vi "Constants.vi"() -> ()   [LabVIEW 2015, in "SLSC-12201 DIO Shared.lvlib"]
doc: "Use this Global VI to access the GUIDs assigned to the page resources of the Custom Device."
uses:
  SLSC-12201 DIO Shared.lvlib
panel:
  in  "Tab Control 2":T1(tab)=enum."Properties"
  in  "GUID Line Page":string="661c9457-bca1-4357-942d-be39bffabc16"
  in  "GUID Port Page":string="b5f9d9e4-a9da-4a9f-991b-22d0b235c7c1"
  in  "GUID EnableDisable Page":string="89b0e4bb-853e-450a-b478-3369bedb40c6"
  in  "GUID Command Page":string="5ef2e5ef-6c3e-41ce-8bf3-8b9cdcedadff"
  in  "GUID Status  Page":string="1b9978d0-bb72-4eda-a9bc-ebfaab5f75ec"
  in  "GUID Outgoing Page":string="c55bf871-3108-4625-9a8c-cf5a91b1839b"
  in  "GUID Incoming Page":string="09713285-c596-431e-bd16-d6aa13349e66"
  in  "GUID Main Page":string="c474772f-1eb5-4c79-98d9-8846819e1c09"
  in  "GUID Channel Interface":string="6ad1a20b-2db8-4c6d-aa6c-0825df07c280"
  in  "Caps Version":string="1.0.0"
  in  "CHM File Name":string="SLSC Module Addon.chm"
  in  "Channel Interface Name":string="Channel Interface"
  in  "Module.Name":string="SLSC-12201"
  in  "product.Num":i32=4098 format="%.0x"
  in  "vendor.Num":i32=4243 format="%.0x"
  in  "CD Version":string="1.0.2"
  in  "Revision A":string="RevA"
  in  "productNumber":string="productNumber"
  in  "vendorNumber":string="vendorNumber"
  in  "capsVersion":string="capsVersion"
  in  "Bank 1":string="Bank 1"
  in  "Input to SLSC":string="Input"
  in  "Chassis Username":string="Chassis Username"
  in  "Command Channel":string="Commands"
  in  "Status Channel":string="Diagnostics"
  in  "Output from SLSC":string="Output"
  in  "Bank 0":string="Bank 0"
  in  "SLSCChannelPath":string="SLSCChannelPath"
  in  "PropertyNames":string="PropertyNames"
  in  "Page Configuration Settings":string="Page Configuration Settings"
  in  "Compiled.Settings":string="Compiled.Settings"
  in  "productNum":string="productNum"
  in  "vendorNum":string="vendorNum"
  in  "Slot CD Processor Affinity":string="Slot CD Processor Affinity"
  in  "SLSC Root CD Version":string="SLSC Root CD Version"
  in  "SLSC Plug-in Paths":string="SLSC Plug-in Paths"
  in  "SLSC Plug-in GUIDs":string="SLSC Plug-in GUIDs"
  in  "SLSC Plug-in Names":string="SLSC Plug-in Names"
  in  "ModuleName":string="ModuleName"
  in  "Module Number":string="Slot #"
  in  "Chassis #":string="Chassis #"
  in  "Chassis IP Address":string="Chassis IP Address"
  in  "SlotX.Property":string="Slot %d.%s"
  in  "Slot CD Name Format":string="Slot %d (%s)"
  in  "Property.Property":string="%s.%s"
  # "(Name needs to match the Module.Name from the device)"
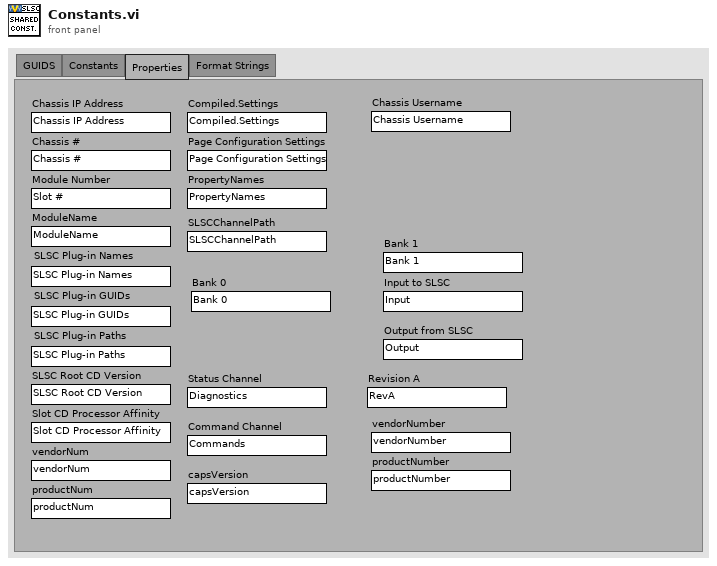
[diagram p1: front panel]
types:
  T1 = enum32{"GUIDS", "Constants", "Properties", "Format Strings"}
diagram:
